vi "H-MEDI Communication and Notice Popup.vi"() -> (0 "HW control on":bool)   [LabVIEW 2019]
doc: "26"
uses:
  <vilib>/Utility/miscctls.llb/LVPointTypeDef.ctl
  <vilib>/Instr/_visa.llb/VISA Configure Serial Port (Instr).vi
panel:
  in  "탭 컨트롤":enum32{"연결", "주의사항"}(tab)
  in  "userContolResourceName":refnum<visa-resource-name>="COM3"
  in  "backPage":bool
  out "연결 상태 확인":bool
  in  "이전":bool
  in  "다음":bool
  out "Notice":string
  in  "주의_backPage":bool
  in  "주의_이전":bool
  in  "주의_다음":bool
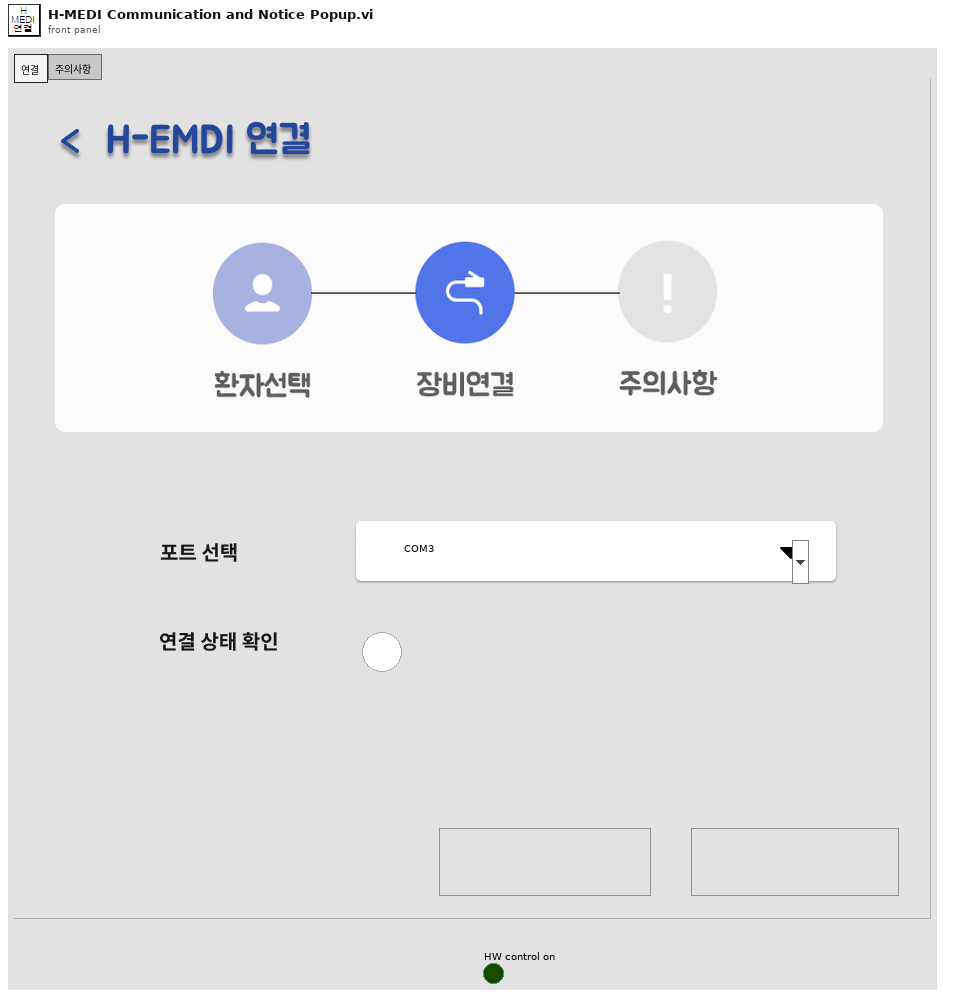
[diagram p1: front panel]
types:
  T1 = typedef "LVPointTypeDef.ctl" = cluster{"Horizontal":i16, "Vertical":i16}
  T2 = cluster{"baud rate (9600)":u32, "flow control (0:none)":u16, "VISA resource name 2":refnum<visa-resource-name>, "termination char\n(0xA = '\\n' = LF) ":u8, "data bits (8)":u16, "parity (0:none)":enum16{"None", "Odd", "Even", "Mark", "Space"}, "timeout (10sec)":u32, "Enable Termination\nChar (T)":bool, "stop bits (10: 1 bit)":u16}
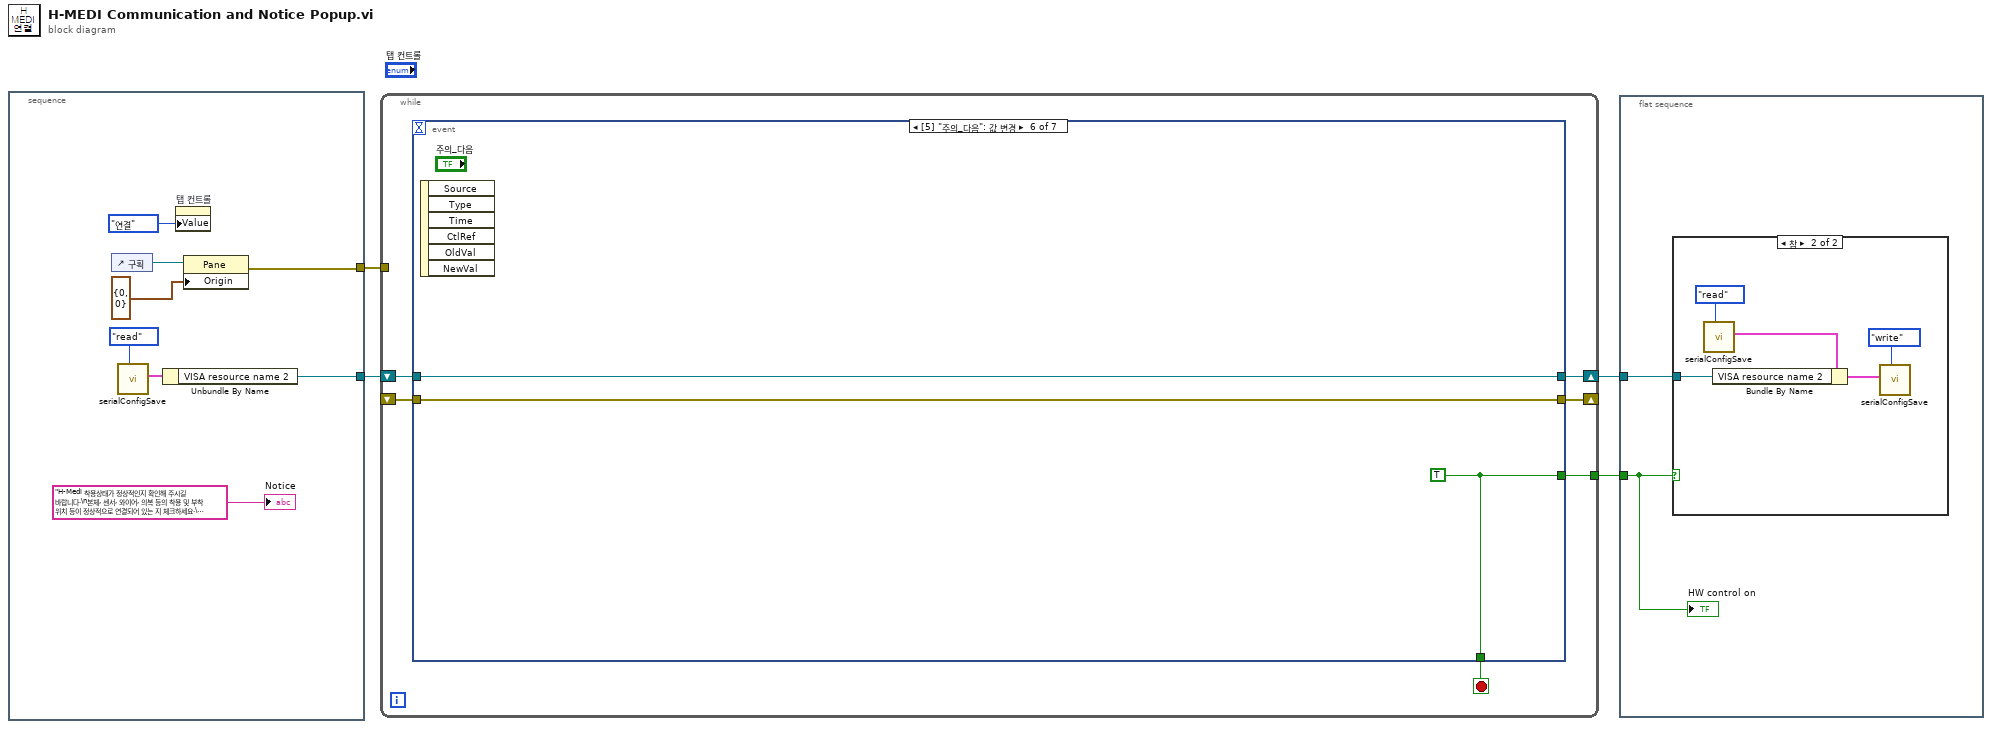
[diagram p0: block diagram]
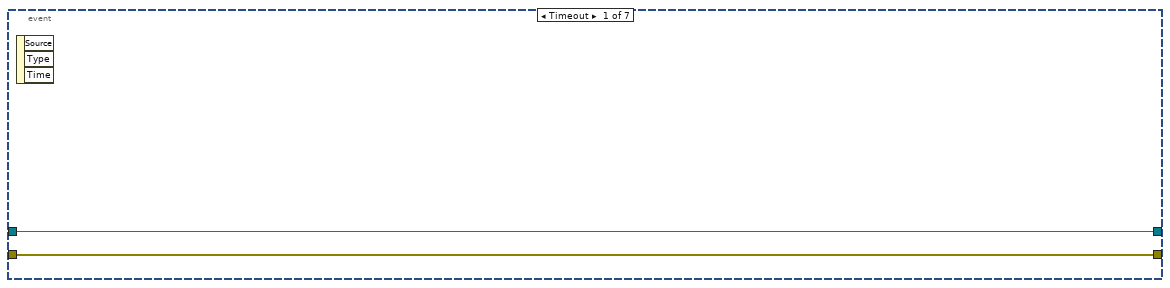
[diagram p3: hidden frame]
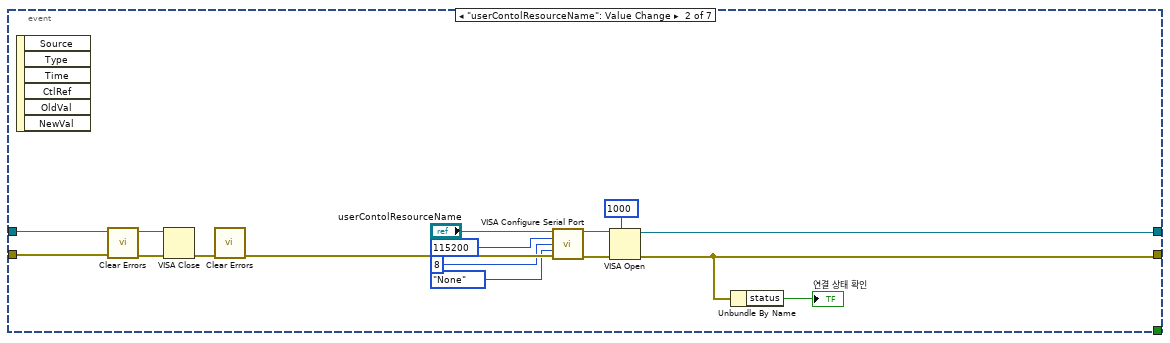
[diagram p4: hidden frame]
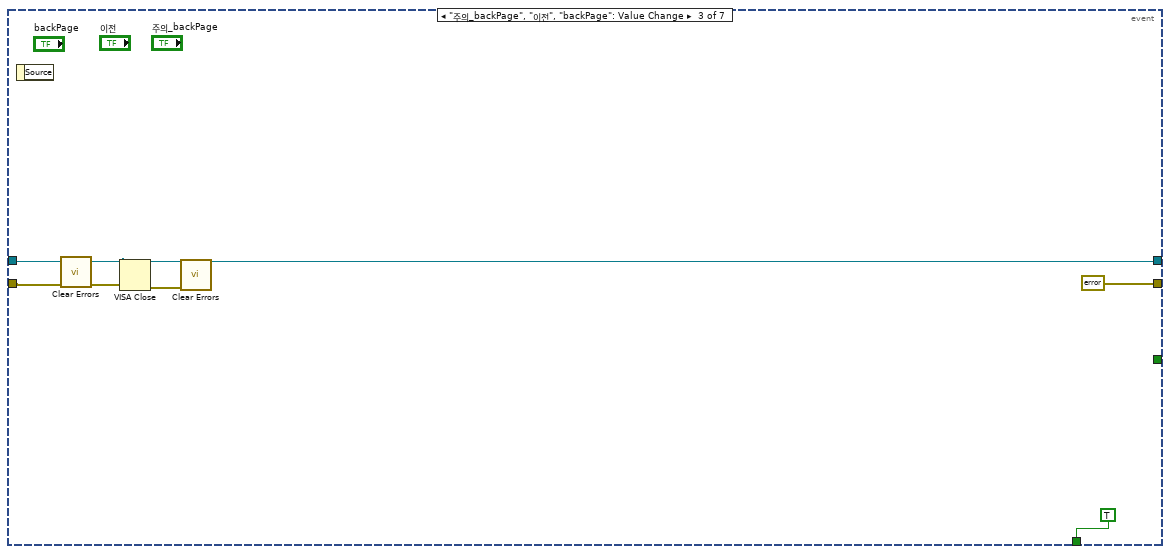
[diagram p5: hidden frame]
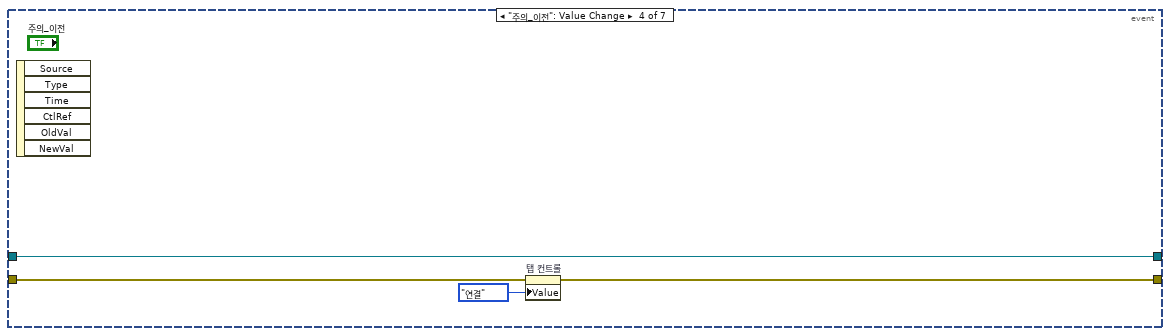
[diagram p6: hidden frame]
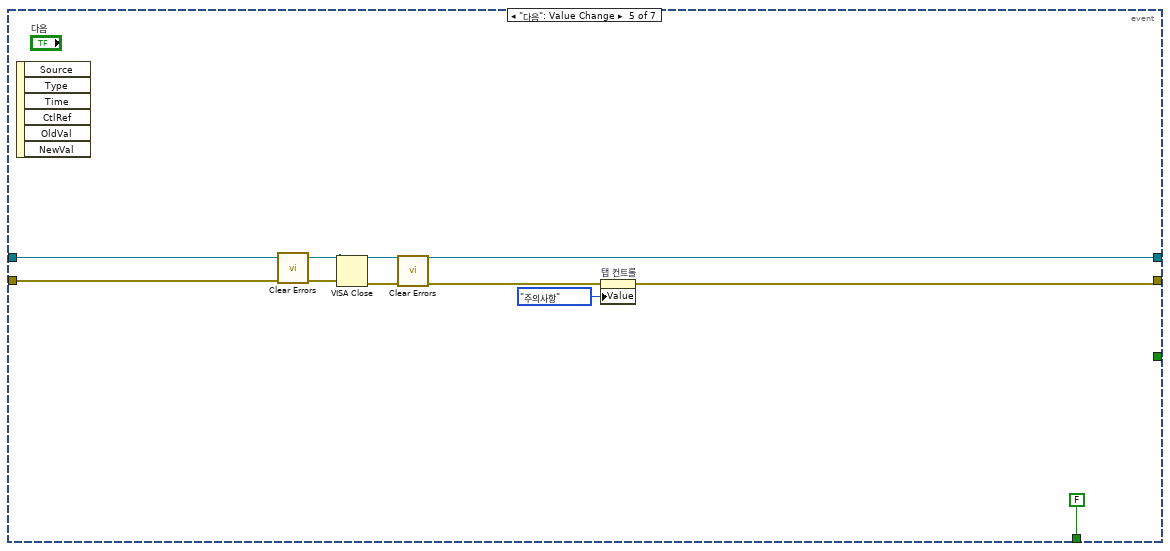
[diagram p7: hidden frame]
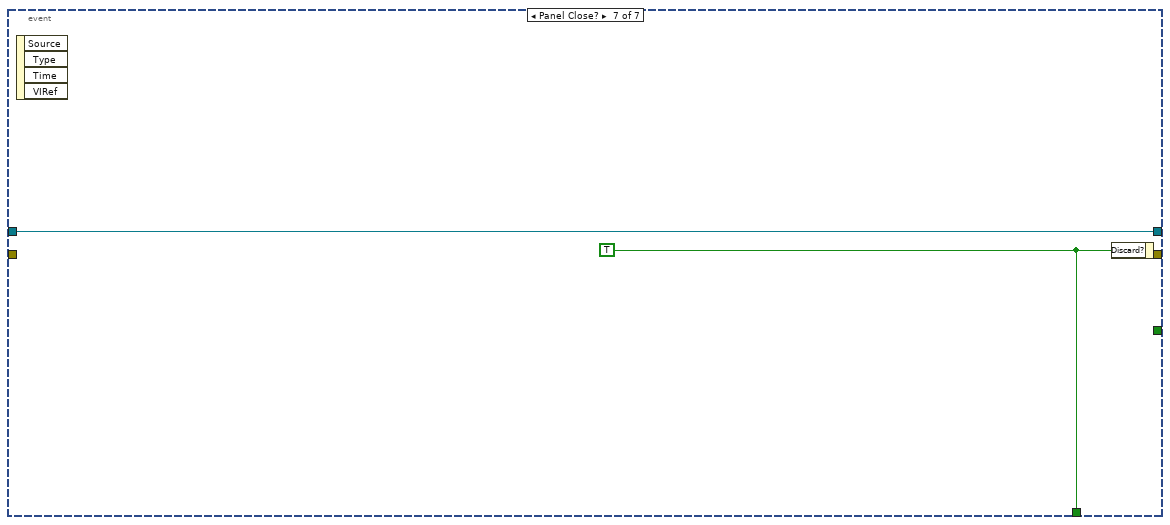
[diagram p8: hidden frame]
diagram:
  n1 = stacked-sequence {
    tunnel: [w10] -> w4
    tunnel: [w6] -> w1
    frame #0 {
      n2 = control-ref of="구획"() -> (w12:refnum<vi>)
      n3 = call "serialConfigSave.vi"("Ctl"=enum16{"read", "write"}."read") -> ("Reurn"=w7:T2)  [unwired: 10 in]
      n4 = Unbundle By Name(w7) -> ("VISA resource name 2"=w6:refnum<visa-resource-name>)
      n5 = property on="탭 컨트롤" class="TabCtl (엄격한)"("Value"=enum32{"연결", "주의사항"}."연결" ("탭 컨트롤")) -> ()  [unwired: 2 in, 2 out]
      n6 = property class="Pane"(reference=w12, "Origin"=T1 {"Horizontal"=0, "Vertical"=0} ("원점")) -> (error out=w10:errorcluster)  [unwired: 1 in, 1 out]
      "Notice" <- "H-Medi 착용상태가 정상적인지 확인해 주시길 바랍니다.\n본체, 센서, 와이어, 의복 등의 착용 및 부착 위치 등이 정상적으로 연결되어 있는 지 체크하세요.\n이후 구동기가 움직일 수 있습니다. 와이어를 손으로 잡지 마세요."
    }
  }
  n7 = while {
    tunnel: w4 -> [_]
    shift-right: [w17] -> _
    shift-left: _ -> [w16]
    shift-right: [w15] -> w3
    shift-left: w1 -> [w14]
    tunnel: [w13] -> w2
    stop <- w18 stop-if-true
    n8 = event shown="[5] \"주의_다음\": 값 변경" {
      selector: _ -> [_ _ _ _ _ _ _]
      dyn-events: _ -> [_ _ _ _ _ _ _]
      timeout: _ -> [_ _ _ _ _ _ _]
      tunnel: [_ _ TRUE _ FALSE w54 w58] -> w18
      tunnel: [w19 w26 errorcluster {"status"=FALSE, "code"=0, "source"=""} ("error out") w42 w47 w55 _] -> w17
      tunnel: w16 -> [w19 w25 w39 w43 w50 w55 _]
      tunnel: [w20 w23 w36 w45 w49 w56 w57] -> w15
      tunnel: w14 -> [w20 w24 w36 w45 w49 w56 w57]
      tunnel: [_ _ _ _ _ w54 _] -> w13
      event Timeout {
        n9 = event-data() -> ()  [unwired: 1 in, 3 out]
      }
      event "userContolResourceName": Value Change {
        n10 = event-data() -> ()  [unwired: 1 in, 6 out]
        n11 = call <vilib>:"Clear Errors.vi"("error in (no error)"=w25) -> ("error out"=w30:errorcluster)  [unwired: 5 in, 1 out]
        n12 = VISA Close(VISA resource name=w24, error in (no error)=w30) -> (error out=w31:errorcluster)
        n13 = call <vilib>:"Clear Errors.vi"("error in (no error)"=w31) -> ("error out"=w32:errorcluster)  [unwired: 5 in, 1 out]
        n14 = call-poly "VISA Configure Serial Port"("VISA resource name"="userContolResourceName", "baud rate (9600)"=u32 115200, "data bits (8)"=u16 8, "parity (0:none)"=enum16{"None", "Odd", "Even", "Mark", "Space"}."None", "error in (no error)"=w32) -> ("VISA resource name out"=w34:refnum<visa-resource-name>, "error out"=w33:errorcluster)  [unwired: 9 in]
        n15 = VISA Open(timeout (0)=u32 1000 ("VISA 열기 타임아웃(0)"), error in (no error)=w33, VISA resource name=w34) -> (VISA resource name=w23:refnum<visa-resource-name>, error out=w26:errorcluster)  [unwired: 2 in]
        n16 = Unbundle By Name(w26) -> ("status"=→"연결 상태 확인":bool)
      }
      event "주의_backPage", "이전", "backPage": Value Change {
        n17 = event-data() -> ()  [unwired: 1 in, 1 out]
        n18 = call <vilib>:"Clear Errors.vi"("error in (no error)"=w39) -> ("error out"=w41:errorcluster)  [unwired: 5 in, 1 out]
        n19 = VISA Close(VISA resource name=w36, error in (no error)=w41) -> (error out=w40:errorcluster)
        n20 = call <vilib>:"Clear Errors.vi"("error in (no error)"=w40) -> ()  [unwired: 5 in, 2 out]
      }
      event "주의_이전": Value Change {
        n21 = event-data() -> ()  [unwired: 1 in, 6 out]
        n22 = property on="탭 컨트롤" class="TabCtl (엄격한)"(error in=w43, "Value"=enum32{"연결", "주의사항"}."연결" ("탭 컨트롤")) -> (error out=w42:errorcluster)  [unwired: 1 in, 1 out]
      }
      event "다음": Value Change {
        n23 = event-data() -> ()  [unwired: 1 in, 6 out]
        n24 = call <vilib>:"Clear Errors.vi"("error in (no error)"=w50) -> ("error out"=w52:errorcluster)  [unwired: 5 in, 1 out]
        n25 = VISA Close(VISA resource name=w49, error in (no error)=w52) -> (error out=w51:errorcluster)
        n26 = call <vilib>:"Clear Errors.vi"("error in (no error)"=w51) -> ("error out"=w48:errorcluster)  [unwired: 5 in, 1 out]
        n27 = property on="탭 컨트롤" class="TabCtl (엄격한)"(error in=w48, "Value"=enum32{"연결", "주의사항"}."주의사항" ("탭 컨트롤")) -> (error out=w47:errorcluster)  [unwired: 1 in, 1 out]
      }
      event "주의_다음": Value Change {
        w54 = TRUE
        n28 = event-data() -> ()  [unwired: 1 in, 6 out]
      }
      event Panel Close? {
        w58 = TRUE
        n29 = event-data() -> ()  [unwired: 1 in, 4 out]
        n30 = event-data("Discard?"=w58) -> ()  [unwired: 1 in, 1 out]
      }
    }
  }
  n31 = flat-sequence {
    tunnel: w3 -> [w59]
    tunnel: w2 -> [w60]
    frame #0 {
      n32 = case shown="참" w60 {
        tunnel: w59 -> [_ w62]
        frame False {
        }
        frame True {
          n33 = call "serialConfigSave.vi"("Ctl"=enum16{"read", "write"}."read") -> ("Reurn"=w63:T2)  [unwired: 10 in]
          n34 = Bundle By Name(cluster=w63, "VISA resource name 2"=w62) -> (w61:T2)
          n35 = call "serialConfigSave.vi"("Ctl"=enum16{"read", "write"}."write", "ViSA Config"=w61) -> ()  [unwired: 9 in, 1 out]
        }
      }
      "HW control on" <- w60
    }
  }
